vi "CAN Config Stress Test.vi"() -> ()   [LabVIEW 2021]
uses:
  Ethernet/Ethernet.lvclass
  Ethernet/Config Types/CAN Settings.ctl
panel:
  out "Iteration":i32
  in  "stop":bool
  out "Read equal?":bool
  out "In == out?":bool
  out "XML written equal?":bool
  out "CAN Settings":T1
  out "Configuration Error?":bool
  out "error out":errorcluster
  in  "UDP port":u16=54321
  in  "TCP port":u16=12345
  in  "Box IP address":string="192.168.1.100"
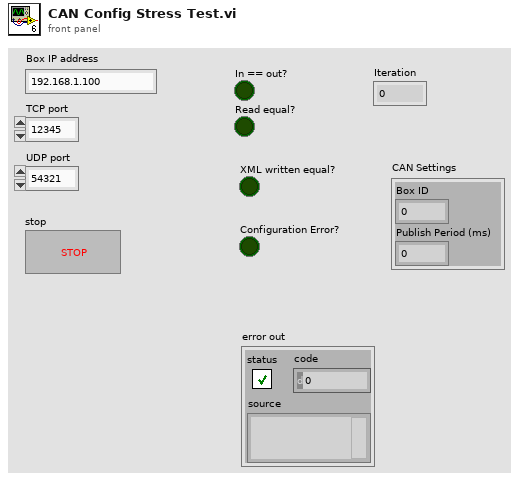
[diagram p1: front panel]
types:
  T1 = typedef "Battery Simulator 1200 LabVIEW Driver.lvlib/Ethernet.lvclass/CAN Settings.ctl" = cluster{"Box ID":i32, "Publish Period (ms)":i32}
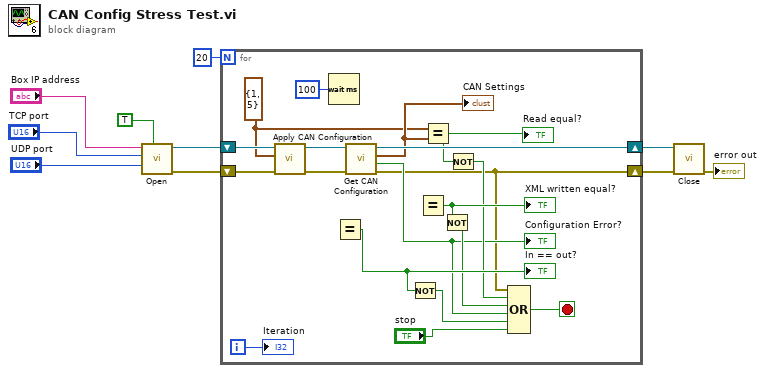
[diagram p0: block diagram]
diagram:
  n1 = call "Open.vi"("Connect for Config Only? (F)"=TRUE, "UDP port"="UDP port", "TCP port"="TCP port", "Box IP address"="Box IP address") -> ("error out"=w10:errorcluster, "ENET out"=w9:refnum<class "Ethernet.lvclass">)  [unwired: 6 in]
  n2 = for {
    N: 20 -> [_]
    shift-right: [w12] -> w3
    shift-left: w10 -> [w29]
    shift-right: [w25] -> w2
    shift-left: w9 -> [w28]
    i -> [w11]
    stop <- w13 stop-if-true
    w23 = T1 {"Box ID"=1, "Publish Period (ms)"=5} ("CAN Settings")
    n3 = call "Apply CAN Configuration.vi"("error in (no error)"=w29, "CAN Settings"=w23, "Ethernet in"=w28) -> ("error out"=w27:errorcluster, "Ethernet out"=w26:refnum<class "Ethernet.lvclass">)  [unwired: 7 in]
    n4 = Wait (ms)(milliseconds to wait=u32 100) -> ()  [unwired: 1 out]
    n5 = Equal?() -> (x = y?=w19:bool)  [unwired: 2 in]
    "In == out?" <- w19
    n6 = call "Get CAN Configuration.vi"("error in (no error)"=w27, "Ethernet in"=w26) -> ("error out"=w12:errorcluster, "Configuration Error?"=w16:bool, "CAN Settings"=w24:T1, "Ethernet out"=w25:refnum<class "Ethernet.lvclass">)  [unwired: 6 in]
    "Configuration Error?" <- w16
    "CAN Settings" <- w24
    n7 = Not(x=w19) -> (.not. x?=w15:bool)
    n8 = Equal?() -> (x = y?=w21:bool)  [unwired: 2 in]
    "XML written equal?" <- w21
    n9 = Equal?(x=w23, y=w24) -> (x = y?=w20:bool)
    "Read equal?" <- w20
    n10 = Not(x=w21) -> (.not. x?=w17:bool)
    n11 = Not(x=w20) -> (.not. x?=w18:bool)
    n12 = Compound Arithmetic op=OR(w12, w18, w17, w16, w15, "stop") -> (w13:bool)
    "Iteration" <- w11
  }
  n13 = call-dynamic "Close.vi"("error in (no error)"=w3, "ENET in"=w2) -> ("error out"=→"error out":errorcluster)  [unwired: 9 in]
